vi "NTJ_OldVer_Get_PersistFlag.vi"(8 "error in (no error)":errorcluster, 11 "Entry Name":string) -> (0 "error out":errorcluster, 3 "PersistFlag":bool)   [LabVIEW 2019]
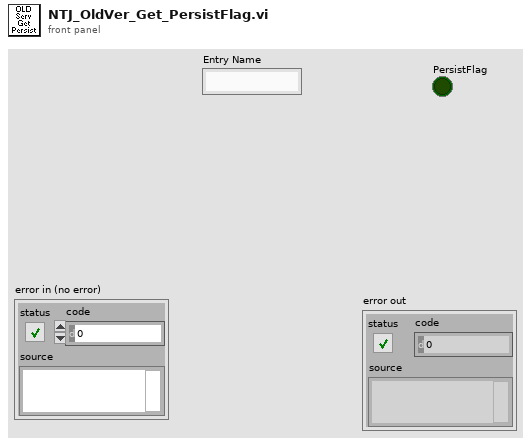
[diagram p1: front panel]
types:
  T1 = typedef "Field Data.ctl" = cluster{"Dbl":dbl, "String":string, "Type":T2, "Boolean":bool, "Sequence #":T3, "Flags":u8}
  T2 = typedef "Field Type.ctl" = enum8{"Invalid", "Bool", "Numeric", "String", "Raw", "Boolean Array", "Numeric Array", "String Array", "RPC"}
  T3 = typedef "Sequence.ctl" = u16
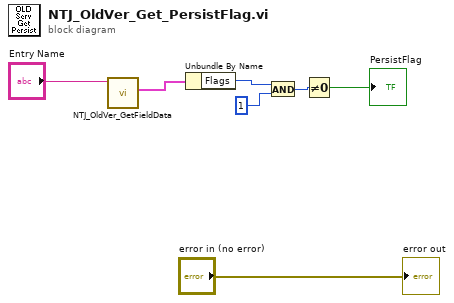
[diagram p0: block diagram]
diagram:
  n1 = call "NTJ_OldVer_GetFieldData.vi"("Entry Name"="Entry Name") -> ("Field Value Out"=w5:T1)  [unwired: 7 in, 2 out]
  n2 = Unbundle By Name(w5) -> ("Flags"=w4:u8)
  n3 = And(x=w4, y=u8 1) -> (x .and. y?=w2:u8)
  n4 = Not Equal To 0?(x=w2) -> (x != 0?=→"PersistFlag":bool)
  "error out" <- "error in (no error)"
